vi "USB_CAN_ABOUT_DLG.vi"(10 "Info":string, 11 "Title":string) -> ()   [LabVIEW 2011]
panel:
  in  "OK":bool
  out "info":string
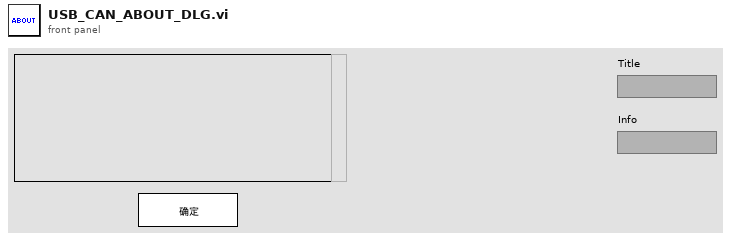
[diagram p1: front panel]
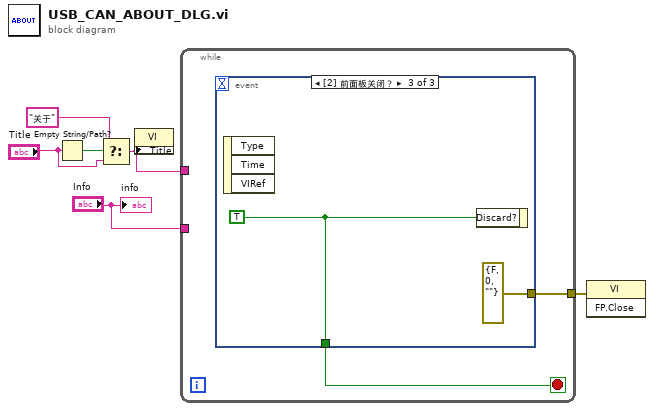
[diagram p0: block diagram]
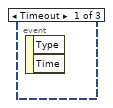
[diagram p2: hidden frame]
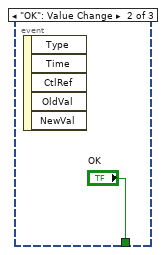
[diagram p3: hidden frame]
diagram:
  n1 = Empty String/Path?(string/path="Title") -> (empty?=w6:bool)
  n2 = Select(t="关于", s=w6, f="Title") -> (s? t:f=w2:string)
  n3 = property class="VI"("Front Panel.Title"=w2) -> ()  [unwired: 2 in, 2 out]
  n4 = while {
    tunnel: "Info" -> [_]
    tunnel: w2 -> [_]
    tunnel: [w7] -> w1
    stop <- w8 stop-if-true
    n5 = event shown="[2] 前面板关闭？" {
      selector: _ -> [_ _ _]
      dyn-events: _ -> [_ _ _]
      timeout: _ -> [_ _ _]
      tunnel: [_ "OK" w11] -> w8
      tunnel: [_ _ errorcluster {"status"=FALSE, "code"=0, "source"=""} ("错误输入（无错误）")] -> w7
      event Timeout {
        n6 = event-data() -> ()  [unwired: 1 in, 2 out]
      }
      event "OK": Value Change {
        n7 = event-data() -> ()  [unwired: 1 in, 5 out]
      }
      event Panel Close? {
        w11 = TRUE ("放弃？")
        n8 = event-data() -> ()  [unwired: 1 in, 3 out]
        n9 = event-data("Discard?"=w11) -> ()  [unwired: 1 in, 1 out]
      }
    }
  }
  n10 = invoke class="VI" method="FP.Close"(error in=w1) -> ()  [unwired: 2 in, 3 out]
  "info" <- "Info"
